vi "FTW-File-AppendStringToFileName.vi"(2 "String":string, 7 "Path In":path) -> (8 "Path Out":path)   [LabVIEW 2015]
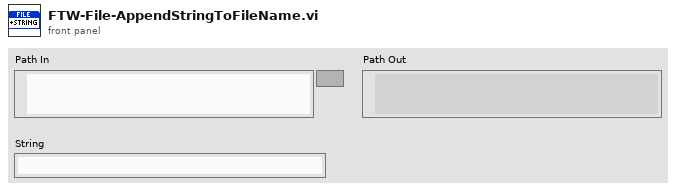
[diagram p1: front panel]
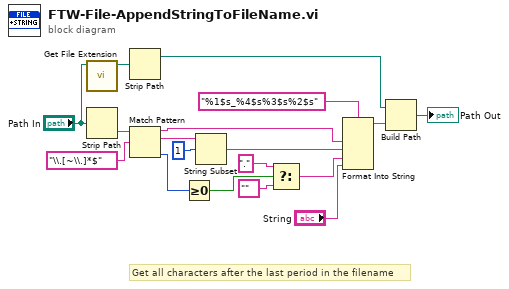
[diagram p0: block diagram]
diagram:
  # "Get all characters after the last period in the filename"
  n1 = call <vilib>:"Get File Extension.vi"("file"="Path In") -> ("dup file"=w16:path)  [unwired: 6 in, 4 out]
  n2 = Strip Path(path="Path In") -> (name=w9:string)  [unwired: 1 out]
  n3 = Strip Path(path=w16) -> (stripped path=w17:path)  [unwired: 1 out]
  n4 = Match Pattern(string=w9, regular expression="\\.[~\\.]*$") -> (before substring=w5:string, match substring=w10:string, offset past match=w4:i32)  [unwired: 2 out]
  n5 = Greater Or Equal To 0?(x=w4) -> (x >= 0?=w13:bool)
  n6 = String Subset(string=w10, offset (0)=1) -> (substring=w3:string)  [unwired: 1 out]
  n7 = Select(t=".", s=w13, f="") -> (s? t:f=w12:string)
  n8 = Format Into String(format string="%1$s_%4$s%3$s%2$s", w5, w3, w12, "String") -> (resulting string=w14:string)  [unwired: 2 in, 1 out]
  n9 = Build Path(base path=w17, name or relative path=w14) -> (appended path=→"Path Out":path)
